vi "replace cursor - plot ref.vi"(4 "cursor state":T1(ring)=enum."boring", 5 "Color Box":u32(colorbox)=327424, 6 "label":enum16{"hide", "show x", "show y", "show (x,y)"}(ring), 7 "action":enum16{"", "read", "write"}(ring)=enum."write", 8 "cursor index":i32, 9 "new  Y":dbl=nan, 10 "new X":dbl=nan, 11 "Plot ref in":refnum<vi>) -> (1 "read Y":dbl, 2 "read X":dbl, 3 "Plot ref out":refnum<vi>)   [LabVIEW 2018]
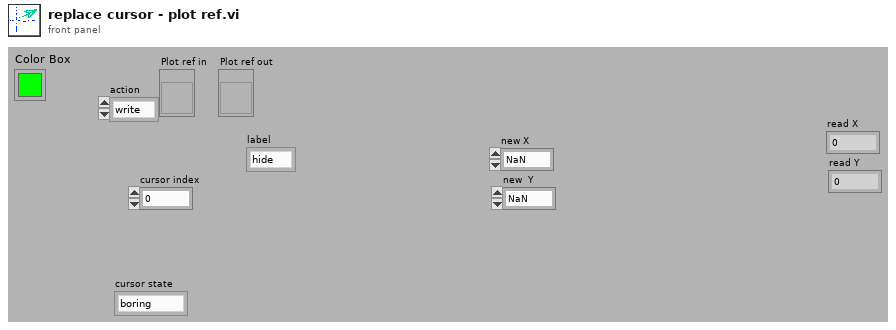
[diagram p1: front panel]
types:
  T1 = enum16{"normal", "alert", "fuzzy", "interesting", "boring", "colored"}
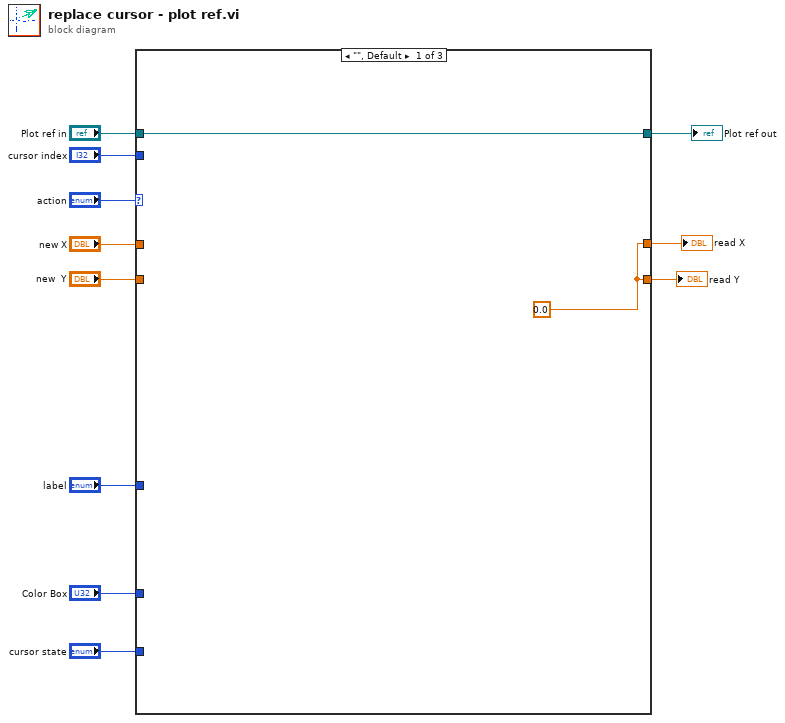
[diagram p0: block diagram]
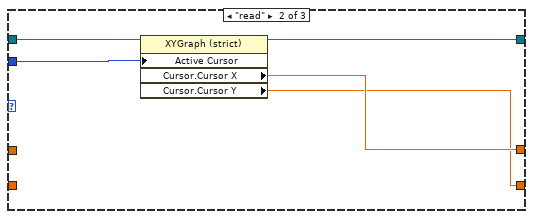
[diagram p2: hidden frame]
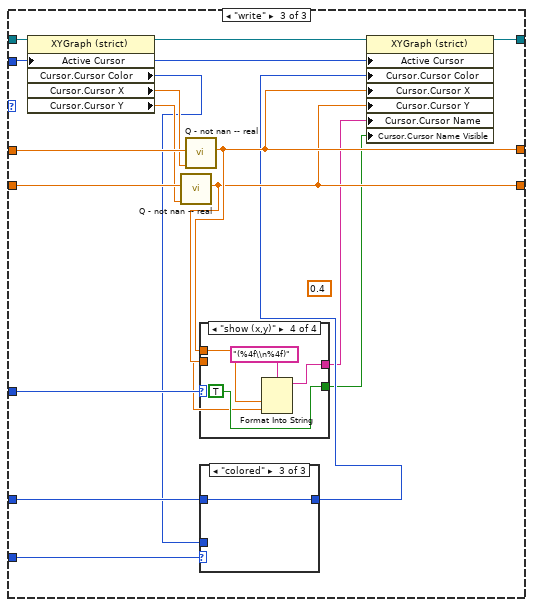
[diagram p3: hidden frame]
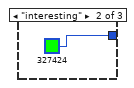
[diagram p5: hidden frame]
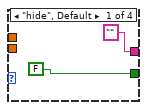
[diagram p6: hidden frame]
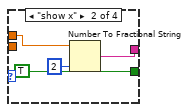
[diagram p7: hidden frame]
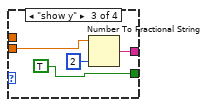
[diagram p8: hidden frame]
diagram:
  n1 = case shown="\"\", Default" "action" {
    tunnel: "new  Y" -> [_ _ w34]
    tunnel: "new X" -> [_ _ w35]
    tunnel: [w13 w17 w27] -> w8
    tunnel: [w13 w16 w26] -> w7
    tunnel: "label" -> [_ _ w33]
    tunnel: "Color Box" -> [_ _ w32]
    tunnel: "cursor state" -> [_ _ w31]
    tunnel: [w12 w18 w22] -> w3
    tunnel: "cursor index" -> [_ w15 w19]
    tunnel: "Plot ref in" -> [w12 w14 w20]
    frame "", Default {
      w13 = 0.0
    }
    frame "read" {
      n2 = property on="Property Node" class="XYGraph (strict)"(reference=w14, "Active Cursor"=w15) -> (reference out=w18:refnum<vi>, "Cursor.Cursor X"=w17:dbl, "Cursor.Cursor Y"=w16:dbl)  [unwired: 1 in, 1 out]
    }
    frame "write" {
      (unwired) 0.4 ("Label Offset.X")
      n3 = property on="Property Node" class="XYGraph (strict)"(reference=w20, "Active Cursor"=w19) -> (reference out=w30:refnum<vi>, "Cursor.Cursor Color"=w21:u32, "Cursor.Cursor X"=w29:dbl, "Cursor.Cursor Y"=w28:dbl)  [unwired: 1 in, 1 out]
      n4 = call "Q - not nan -- real.vi"("default"=w28, "Numeric"=w34) -> ("out"=w26:dbl)  [unwired: 8 in, 1 out]
      n5 = call "Q - not nan -- real.vi"("default"=w29, "Numeric"=w35) -> ("out"=w27:dbl)  [unwired: 8 in, 1 out]
      n6 = case shown="\"show (x,y)\"" w33 {
        tunnel: w27 -> [_ w44 _ w50]
        tunnel: ["" ("format string") w43 w47 w53] -> w24
        tunnel: [FALSE ("Name Visible") TRUE ("Name Visible") TRUE ("Name Visible") TRUE ("Name Visible")] -> w23
        tunnel: w26 -> [_ _ w46 w49]
        frame "hide", Default {
        }
        frame "show x" {
          n7 = Number To Fractional String(number=w44, precision (6)=i16 2) -> (F-format string=w43:string)  [unwired: 2 in]
        }
        frame "show y" {
          n8 = Number To Fractional String(number=w46, precision (6)=i16 2) -> (F-format string=w47:string)  [unwired: 2 in]
        }
        frame "show (x,y)" {
          n9 = Format Into String(format string="(%4f\\n%4f)", w50, w49) -> (resulting string=w53:string)  [unwired: 2 in, 1 out]
        }
      }
      n10 = case shown="\"colored\"" w31 {
        tunnel: [w36 u32 327424 ("Color Box") w38] -> w25
        tunnel: w32 -> [_ _ w38]
        tunnel: w21 -> [w36 _ _]
        frame "boring", Default {
        }
        frame "interesting" {
        }
        frame "colored" {
        }
      }
      n11 = property on="Property Node" class="XYGraph (strict)"(reference=w30, "Active Cursor"=w19, "Cursor.Cursor Color"=w25, "Cursor.Cursor X"=w27, "Cursor.Cursor Y"=w26, "Cursor.Cursor Name"=w24, "Cursor.Cursor Name Visible"=w23) -> (reference out=w22:refnum<vi>)  [unwired: 1 in, 1 out]
    }
  }
  "read X" <- w8
  "read Y" <- w7
  "Plot ref out" <- w3
